vi "Find baseplate center.vi"() -> ()   [LabVIEW 2018]
uses:
  Classes/Workspace/Carrier Tray/Assembly Tray.lvclass
  Classes/Controller/Controller.lvclass
  Classes/Workspace/Workspace.ctl
  Classes/Workspace/Fixture.lvclass
panel:
  out "error out":errorcluster
  in  "error in (no error)":errorcluster
  out "Workspace":T1
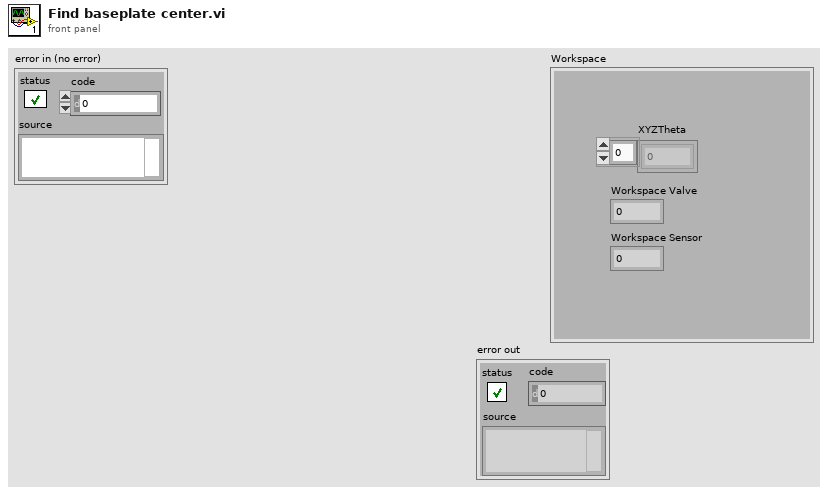
[diagram p1: front panel]
types:
  T1 = typedef "Fixture.lvclass/Workspace.ctl" = cluster{"XYZTheta":dbl[], "Workspace Valve":i32, "Workspace Sensor":i32}
  T2 = typedef "Controller.lvclass/Controllers.ctl" = cluster{"I-O.lvclass":refnum<class "I-O.lvclass">, "Gantry":refnum<k24>, "Dispenser":refnum<visa-resource-name>}
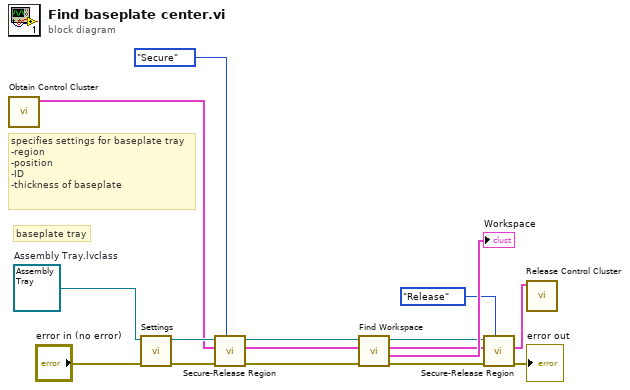
[diagram p0: block diagram]
diagram:
  w16 = refnum<class "Assembly Tray.lvclass"> refnum  # Assembly Tray.lvclass
  # "specifies settings for baseplate tray\n-region\n-position\n-ID \n-thickness of baseplate"
  # "baseplate tray"
  n1 = call "Obtain Control Cluster.vi"() -> ("Control Out"=w12:T2)  [unwired: 11 in]
  n2 = call-dynamic "Settings.vi"("error in (no error)"="error in (no error)", "Assembly Tray In"=w16) -> ("error out"=w6:errorcluster, "Assembly Tray Out"=w14:refnum<class "Assembly Tray.lvclass">)  [unwired: 8 in]
  n3 = call-dynamic "Secure-Release Region.vi"("Action"=enum16{"Secure", "Release"}."Secure", "error in (no error)"=w6, "Control In"=w12, "Carrier Tray in"=w14) -> ("error out"=w5:errorcluster, "Control Out"=w11:T2, "Carrier Tray out"=w13:refnum<class "Assembly Tray.lvclass">)  [unwired: 5 in]
  n4 = call-dynamic "Find Workspace.vi"("Error In"=w5, "Control In"=w11, "Carrier Tray in"=w13) -> ("Error Out"=w4:errorcluster, "Workspace"=→"Workspace":T1, "Control Out"=w10:T2, "Carrier Tray Out"=w8:refnum<class "Assembly Tray.lvclass">)  [unwired: 5 in]
  n5 = call-dynamic "Secure-Release Region.vi"("Action"=enum16{"Secure", "Release"}."Release", "error in (no error)"=w4, "Control In"=w10, "Carrier Tray in"=w8) -> ("error out"=→"error out":errorcluster, "Control Out"=w9:T2)  [unwired: 5 in, 1 out]
  n6 = call "Release Control Cluster.vi"("output cluster"=w9) -> ()  [unwired: 11 in]
